vi "KnownTagsFGV.vi"(7 "Tag Cmd":T1, 8 "error in (no error)":errorcluster, 9 "ini Path":path=path "E:/Mark's Data/OneDrive/Documents/LabVIEW Projects/ComicCleaner/Main.vi", 11 "New Tag":string) -> (0 "error out":errorcluster, 3 "Known Tags":string[](array[string]))   [LabVIEW 2022 SP3]
uses:
  TypeDefs/Tag Cmd.ctl
  <vilib>/Utility/config.llb/Write Key (Boolean).vi
  <vilib>/Utility/config.llb/NI_LVConfig.lvlib
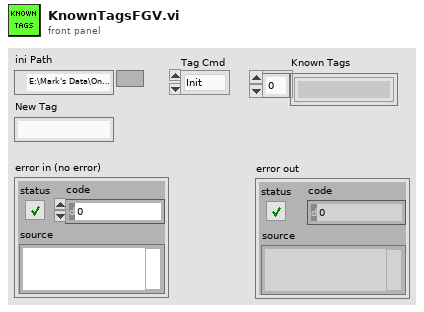
[diagram p1: front panel]
types:
  T1 = typedef "Tag Cmd.ctl" = enum16{"Init", "Get Known", "Set Known"}
  T2 = typedef "NI_LVConfig.lvlib/Config Data RefNum.ctl" = refnum<k1>
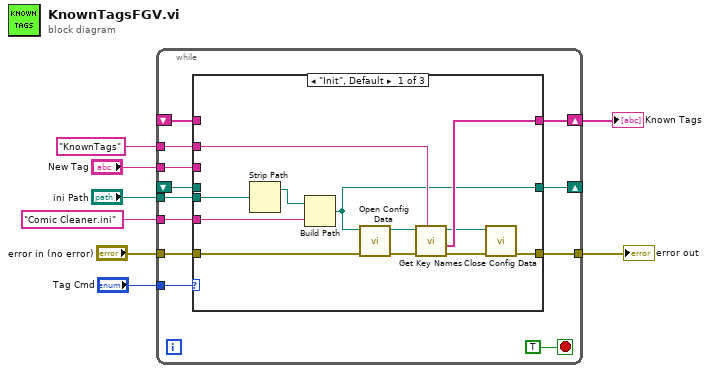
[diagram p0: block diagram]
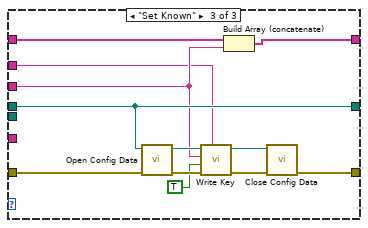
[diagram p3: hidden frame]
diagram:
  n1 = while {
    tunnel: "Tag Cmd" -> [w20]
    shift-right: [w14] -> w7
    shift-left: _ -> [w11]
    tunnel: "error in (no error)" -> [w18]
    tunnel: "ini Path" -> [w17]
    tunnel: "Comic Cleaner.ini" -> [w16]
    tunnel: "KnownTags" ("section") -> [w15]
    tunnel: [w13] -> w2
    shift-right: [w12] -> _
    shift-left: _ -> [w10]
    tunnel: "New Tag" -> [w9]
    stop <- TRUE stop-if-true
    n2 = case shown="\"Init\", Default" w20 {
      tunnel: w18 -> [w32 w33 w47]
      tunnel: w17 -> [w29 _ _]
      tunnel: w16 -> [w31 _ _]
      tunnel: w15 -> [w26 _ w36]
      tunnel: [w25 w35 w44] -> w14
      tunnel: [w22 w33 w37] -> w13
      tunnel: [w21 w34 w46] -> w12
      tunnel: w11 -> [_ w35 w45]
      tunnel: w10 -> [_ w34 w46]
      tunnel: w9 -> [_ _ w41]
      frame "Init", Default {
        n3 = Strip Path(path=w29) -> (stripped path=w30:path)  [unwired: 1 out]
        n4 = Build Path(base path=w30, name or relative path=w31) -> (appended path=w21:path)
        n5 = call <vilib>:"Open Config Data.vi"("error in (no error)"=w32, "configuration file path"=w21) -> ("error out"=w28:errorcluster, "refnum"=w27:T2)  [unwired: 7 in, 1 out]
        n6 = call <vilib>:"Get Key Names.vi"("section"=w26, "error in (no error)"=w28, "refnum"=w27) -> ("error out"=w23:errorcluster, "key names"=w25:string[], "refnum out"=w24:T2)  [unwired: 5 in, 1 out]
        n7 = call <vilib>:"Close Config Data.vi"("error in (no error)"=w23, "refnum"=w24) -> ("error out"=w22:errorcluster)  [unwired: 8 in, 1 out]
      }
      frame "Get Known" {
      }
      frame "Set Known" {
        n8 = call <vilib>:"Open Config Data.vi"("error in (no error)"=w47, "configuration file path"=w46) -> ("error out"=w43:errorcluster, "refnum"=w42:T2)  [unwired: 7 in, 1 out]
        n9 = call-poly <vilib>:"Write Key.vi"("section"=w36, "error in (no error)"=w43, "value"=TRUE, "key"=w41, "refnum"=w42) -> ("error out"=w39:errorcluster, "refnum out"=w38:T2)  [unwired: 4 in, 1 out]
        n10 = Build Array (concatenate)(w45, w41) -> (w44:string[])
        n11 = call <vilib>:"Close Config Data.vi"("error in (no error)"=w39, "refnum"=w38) -> ("error out"=w37:errorcluster)  [unwired: 8 in, 1 out]
      }
    }
  }
  "Known Tags" <- w7
  "error out" <- w2
